vi "BiClient-10.vi"() -> ()   [LabVIEW 2024]
doc: "Demonstrates how to open a connection to a specified host and port, read the data being sent to the port, and display the data on a chart. This VI is designed to stop if the TCP connection is terminated.\n\n<B>Note:</B> Requires the Simple Data Server.vi located in the same library as this VI."
panel:
  in  "# of Points":i32=200
  in  "Function":u16(ring) items=["Random", "Sine wave", "Chirp Pattern"]
  in  "stop":bool
  out "chart":dbl[](graph)
  in  "Address":string="localhost"
  in  "Port":u16=2055 min=1025 step=1
  # "Instructions:\n1. Open the Simple Data\n    Server.vi and run it\n    first.\n2. Run this VI."
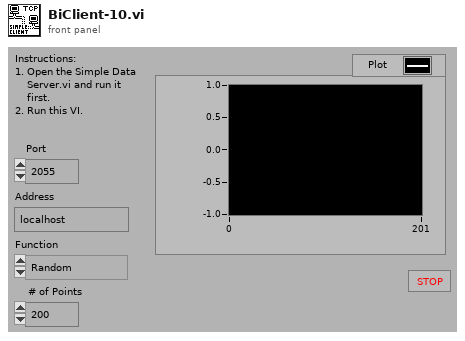
[diagram p1: front panel]
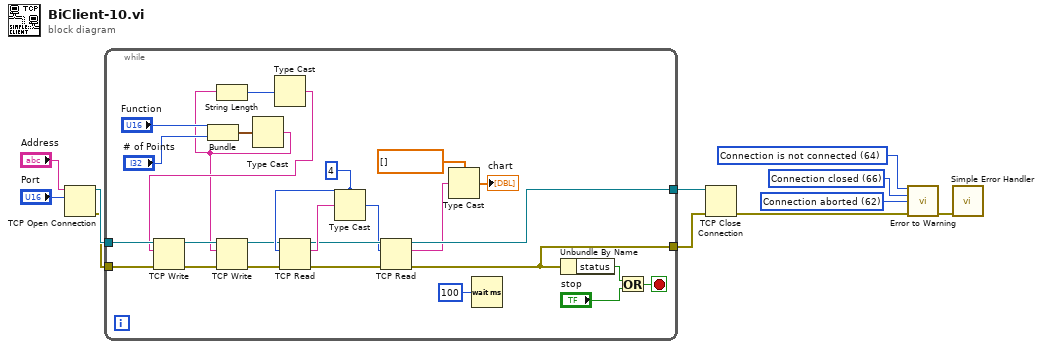
[diagram p0: block diagram]
diagram:
  w1 = 62 items=["No Error", "Argument Error", "Memory Full", "Out of Zone", "End of File", "File Already Open", "Generic File IO Error", "File Not Found", "File Permission Error", "Disk Full", "Duplicate Path", "Too Many Files Open", "Not Enabled", "Resource File Not Found", "Cannot Add Resource", "Resource Not Found", "Image Not Found", "Image Memory Error", "Pen Does Not Exist", "Config Bad Type", "Config Token Not Found", "Config Parse Error", "Config Memory Error", "Bad External Code Format", "Bad External Code Offset", "External Code Not Present", "Null Window", "Destroy Window Mixup", "Null Menu", "Print Aborted", "Bad Print Record", "Print Driver Error", "Windows Error During Print", "Memory Error During Print", "Print Dialog Error", "Generic Print Error", "Invalid Device Refnum", "Device Not Found", "Device Parameter Error", "Device Unit Error", "Can't Open Device", "Device Call Aborted", "Generic Error", "Cancelled By User", "Object ID Too Low", "Object ID Too High", "Object Not In Heap", "Unknown Heap", "Bad DefProc ID", "DefProc Not In Table", "Message Out Of Range", "Null Method", "Unknown Message", "Manager Call Not Supported", "Bad address", "Connection In progress", "Connection timed out", "Connection is already in progress", "Network attribute not supported", "Network error", "Address in use", "System out of memory", "Connection aborted", "Connection refused", "Connection is not connected", "Connection is already connected", "Connection closed", "Initialize error (interapplication manager)", "Bad occurrence", "Wait on unbound occurrence handler", "Occurrence queue overflow", "Bad path", "Semaphore not signaled", "Unrecognized type (interapplication manager)"] ("1st Error to Convert")
  w2 = 66 items=["No Error", "Argument Error", "Memory Full", "Out of Zone", "End of File", "File Already Open", "Generic File IO Error", "File Not Found", "File Permission Error", "Disk Full", "Duplicate Path", "Too Many Files Open", "Not Enabled", "Resource File Not Found", "Cannot Add Resource", "Resource Not Found", "Image Not Found", "Image Memory Error", "Pen Does Not Exist", "Config Bad Type", "Config Token Not Found", "Config Parse Error", "Config Memory Error", "Bad External Code Format", "Bad External Code Offset", "External Code Not Present", "Null Window", "Destroy Window Mixup", "Null Menu", "Print Aborted", "Bad Print Record", "Print Driver Error", "Windows Error During Print", "Memory Error During Print", "Print Dialog Error", "Generic Print Error", "Invalid Device Refnum", "Device Not Found", "Device Parameter Error", "Device Unit Error", "Can't Open Device", "Device Call Aborted", "Generic Error", "Cancelled By User", "Object ID Too Low", "Object ID Too High", "Object Not In Heap", "Unknown Heap", "Bad DefProc ID", "DefProc Not In Table", "Message Out Of Range", "Null Method", "Unknown Message", "Manager Call Not Supported", "Bad address", "Connection In progress", "Connection timed out", "Connection is already in progress", "Network attribute not supported", "Network error", "Address in use", "System out of memory", "Connection aborted", "Connection refused", "Connection is not connected", "Connection is already connected", "Connection closed", "Initialize error (interapplication manager)", "Bad occurrence", "Wait on unbound occurrence handler", "Occurrence queue overflow", "Bad path", "Semaphore not signaled", "Unrecognized type (interapplication manager)"] ("1st Error to Convert")
  w3 = 64 items=["No Error", "Argument Error", "Memory Full", "Out of Zone", "End of File", "File Already Open", "Generic File IO Error", "File Not Found", "File Permission Error", "Disk Full", "Duplicate Path", "Too Many Files Open", "Not Enabled", "Resource File Not Found", "Cannot Add Resource", "Resource Not Found", "Image Not Found", "Image Memory Error", "Pen Does Not Exist", "Config Bad Type", "Config Token Not Found", "Config Parse Error", "Config Memory Error", "Bad External Code Format", "Bad External Code Offset", "External Code Not Present", "Null Window", "Destroy Window Mixup", "Null Menu", "Print Aborted", "Bad Print Record", "Print Driver Error", "Windows Error During Print", "Memory Error During Print", "Print Dialog Error", "Generic Print Error", "Invalid Device Refnum", "Device Not Found", "Device Parameter Error", "Device Unit Error", "Can't Open Device", "Device Call Aborted", "Generic Error", "Cancelled By User", "Object ID Too Low", "Object ID Too High", "Object Not In Heap", "Unknown Heap", "Bad DefProc ID", "DefProc Not In Table", "Message Out Of Range", "Null Method", "Unknown Message", "Manager Call Not Supported", "Bad address", "Connection In progress", "Connection timed out", "Connection is already in progress", "Network attribute not supported", "Network error", "Address in use", "System out of memory", "Connection aborted", "Connection refused", "Connection is not connected", "Connection is already connected", "Connection closed", "Initialize error (interapplication manager)", "Bad occurrence", "Wait on unbound occurrence handler", "Occurrence queue overflow", "Bad path", "Semaphore not signaled", "Unrecognized type (interapplication manager)"] ("1st Error to Convert")
  n1 = TCP Open Connection(address="Address", remote port or service name="Port") -> (connection ID=w7:refnum<k5>, error out=w6:errorcluster)  [unwired: 3 in]
  n2 = while {
    tunnel: w6 -> [w17]
    tunnel: w7 -> [w20]
    tunnel: [w33] -> w8
    tunnel: [w31] -> w9
    stop <- w28 stop-if-true
    w21 = 4
    n3 = Bundle("Function"="Function", "# of Points"="# of Points") -> (w22:cluster{"Function":u16, "# of Points":i32})  [unwired: 1 in]
    n4 = Type Cast(x=w22) -> (*(type *) &x=w12:string)  [unwired: 1 in]
    n5 = String Length(string=w12) -> (length=w13:i32)
    n6 = Type Cast(x=w13) -> (*(type *) &x=w14:string)  [unwired: 1 in]
    n7 = TCP Write(connection ID=w20, data in=w14, error in (no error)=w17) -> (connection ID out=w19:refnum<k5>, error out=w16:errorcluster)  [unwired: 1 in, 1 out]
    n8 = TCP Write(connection ID=w19, data in=w12, error in (no error)=w16) -> (connection ID out=w18:refnum<k5>, error out=w15:errorcluster)  [unwired: 1 in, 1 out]
    n9 = TCP Read(connection ID=w18, bytes to read=w21, error in (no error)=w15) -> (connection ID out=w36:refnum<k5>, data out=w37:string, error out=w35:errorcluster)  [unwired: 2 in]
    n10 = Type Cast(type=w21, x=w37) -> (*(type *) &x=w34:i32)
    n11 = TCP Read(connection ID=w36, bytes to read=w34, error in (no error)=w35) -> (connection ID out=w33:refnum<k5>, data out=w32:string, error out=w31:errorcluster)  [unwired: 2 in]
    n12 = Type Cast(type=dbl[] [] ("chart"), x=w32) -> (*(type *) &x=→"chart":dbl[])
    n13 = Wait (ms)(milliseconds to wait=u32 100) -> ()  [unwired: 1 out]
    n14 = Unbundle By Name(w31) -> ("status"=w30:bool)
    n15 = Or(x=w30, y="stop") -> (x .or. y?=w28:bool)
  }
  n16 = TCP Close Connection(connection ID=w8, error in (no error)=w9) -> (error out=w5:errorcluster)  [unwired: 1 in, 1 out]
  n17 = call <vilib>:"Error to Warning.vi"("1st Error to Convert"=w3, "2nd Error to Convert"=w2, "3rd Error to Convert"=w1, "error in"=w5) -> ("warning out"=w4:errorcluster)  [unwired: 11 in]
  n18 = call <vilib>:"Simple Error Handler.vi"("error in (no error)"=w4) -> ()  [unwired: 4 in, 5 out]
